vi "Hoan_chinh.vi"() -> ()   [LabVIEW 2024]
uses:
  <vilib>/DAQmx/read.llb/DAQmx Read (Analog 1D Wfm NChan 1Samp).vi
  <vilib>/DAQmx/create/channels.llb/DAQmx Create Channel (AI-Voltage-Basic).vi
  <vilib>/DAQmx/configure/timing.llb/DAQmx Timing (Sample Clock).vi
  <vilib>/DAQmx/miscellaneous.llb/DAQmx Fill In Error Info.vi
panel:
  in  "HWSerialNum":i32
  in  "MG17Motor":refnum<k7>(container)
  out "pfPosition":sgl
  out "data":waveform(dbl)[](array[waveform])
  out "Waveform Chart 2":dynamicdata(graph)
  in  "DAQmx Physical Channel":tag
  in  "STOP":bool
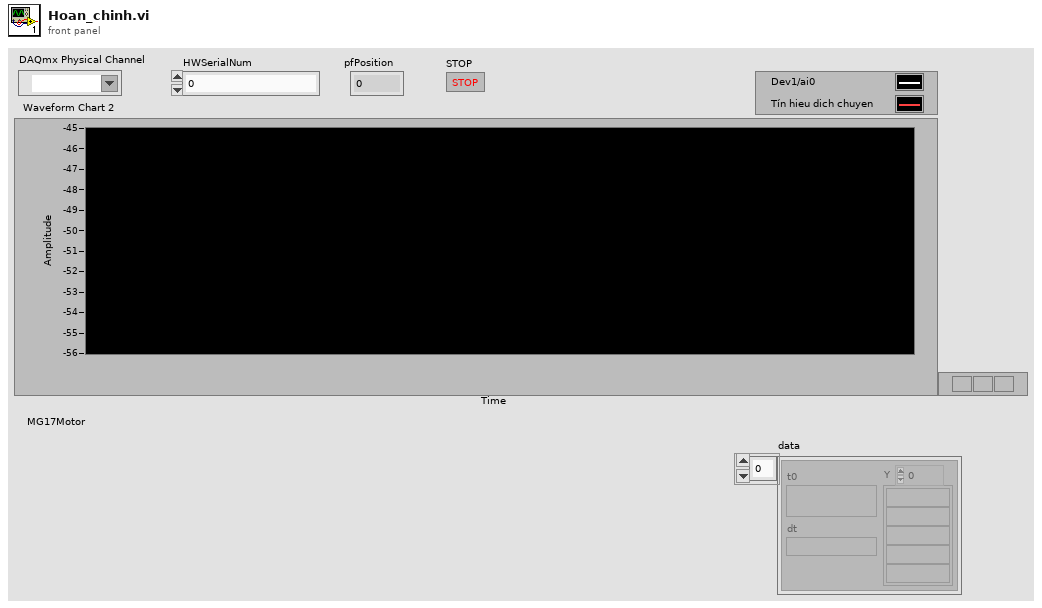
[diagram p1: front panel]
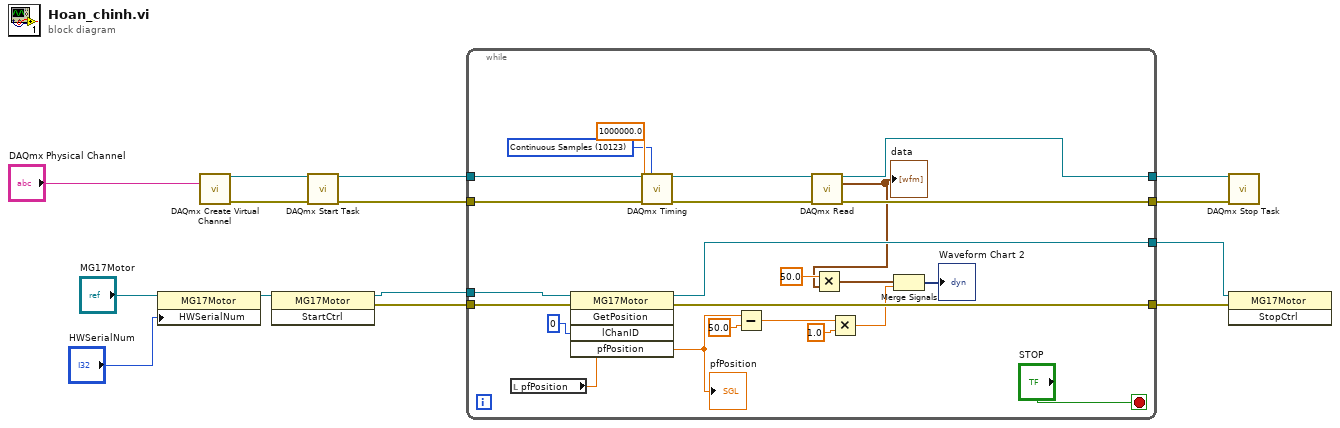
[diagram p0: block diagram]
diagram:
  n1 = property class="MG17Motor"(reference="MG17Motor", "HWSerialNum"="HWSerialNum") -> (reference out=w6:refnum<k7>)  [unwired: 1 in, 1 out]
  n2 = call-poly <vilib>:"DAQmx Create Virtual Channel.vi"("physical channels"="DAQmx Physical Channel") -> ("task out"=w14:refnum<k21>, "error out"=w12:errorcluster)  [unwired: 13 in]
  n3 = invoke class="MG17Motor" method="StartCtrl"(reference=w6) -> (reference out=w5:refnum<k7>, error out=w4:errorcluster)  [unwired: 2 in, 1 out]
  n4 = call <vilib>:"DAQmx Start Task.vi"("task/channels in"=w14, "error in"=w12) -> ("task out"=w13:refnum<k21>, "error out"=w11:errorcluster)  [unwired: 12 in]
  n5 = while {
    tunnel: w13 -> [w20]
    tunnel: w11 -> [w18]
    tunnel: [w37] -> w10
    tunnel: w5 -> [w31]
    tunnel: w4 -> [w30]
    tunnel: [w29] -> w3
    tunnel: [w28] -> w2
    tunnel: [w25] -> w1
    stop <- "STOP" stop-if-true
    w15 = 10123 items=["Finite Samples"=10178, "Continuous Samples"=10123, "Hardware Timed Single Point"=12522] ("sample mode")
    n6 = local read "pfPosition"() -> (w24:sgl)
    n7 = invoke class="MG17Motor" method="GetPosition"(reference=w31, error in=w30, "lChanID"=0, "pfPosition"=w24) -> (reference out=w29:refnum<k7>, error out=w28:errorcluster, "pfPosition"=w27:sgl)  [unwired: 1 in, 2 out]
    "pfPosition" <- w27
    n8 = call-poly <vilib>:"DAQmx Timing.vi"("task/channels in"=w20, "sample mode"=w15, "rate"=1000000.0, "error in"=w18) -> ("task out"=w19:refnum<k21>, "error out"=w17:errorcluster)  [unwired: 10 in]
    n9 = Subtract(x=w27, y=sgl 50.0) -> (x-y=w32:sgl)
    n10 = call-poly <vilib>:"DAQmx Read.vi"("task/channels in"=w19, "error in"=w17) -> ("task out"=w25:refnum<k21>, "data"=w21:waveform(dbl)[], "error out"=w37:errorcluster)  [unwired: 11 in]
    "data" <- w21
    n11 = Multiply(x=50.0, y=w21) -> (x*y=w23:waveform(dbl)[])
    n12 = Multiply(x=w32, y=sgl 1.0 ("x")) -> (x*y=w26:sgl)
    n13 = Merge Signals(w23, w26) -> (→"Waveform Chart 2":dynamicdata)
  }
  n14 = call <vilib>:"DAQmx Stop Task.vi"("task/channels in"=w1, "error in"=w10) -> ()  [unwired: 12 in, 2 out]
  n15 = invoke class="MG17Motor" method="StopCtrl"(reference=w3, error in=w2) -> ()  [unwired: 1 in, 3 out]
